vi "giveSolutionRubix.vi"() -> (1 "Commands to Execute":string[](array[string]))   [LabVIEW 2019]
uses:
  rubix solve code/Rubik's Solver.dll
panel:
  in  "RubixTab solver control":string[][](array[string])
  out "Loesung":i32[](array[numeric])
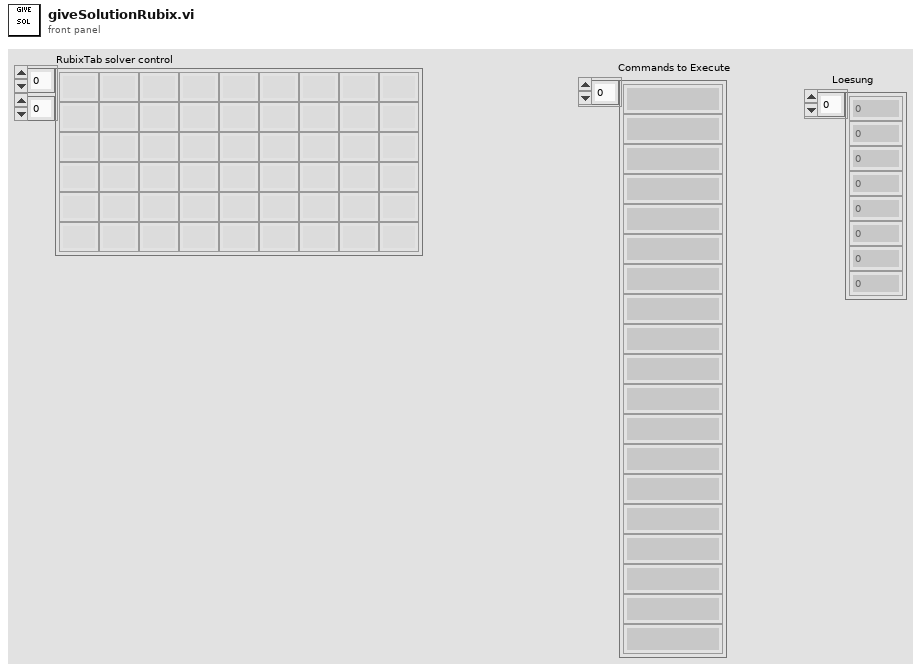
[diagram p1: front panel]
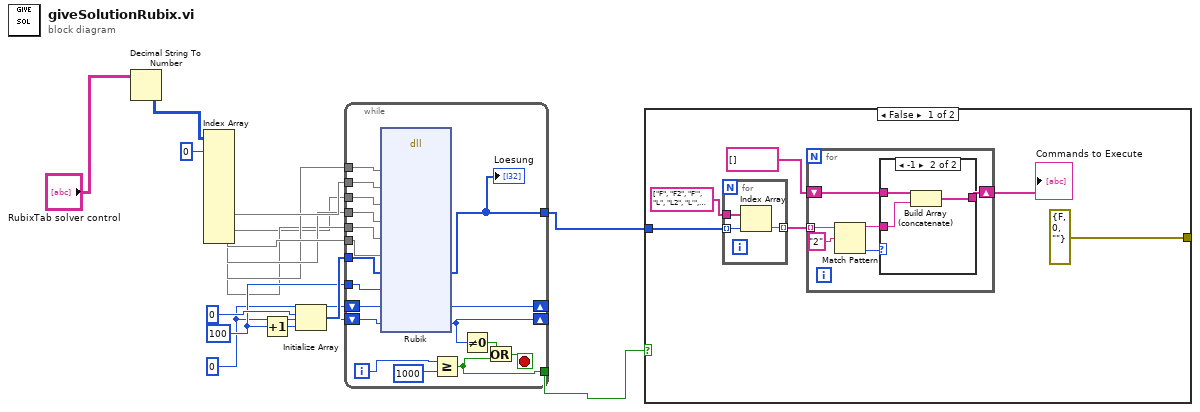
[diagram p0: block diagram]
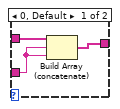
[diagram p2: hidden frame]
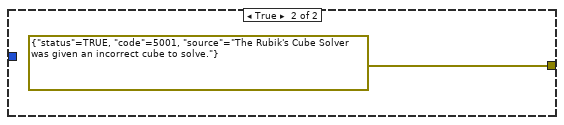
[diagram p3: hidden frame]
diagram:
  w12 = u8 0
  w13 = u16 100
  n1 = Decimal String To Number(string="RubixTab solver control") -> (number=w2:i32[][])  [unwired: 2 in, 1 out]
  n2 = Index Array(array=w2, index (row) #1=0 ("disabled index (col)")) -> (element #1=w10:i32[], element #2=w5:i32[], element #3=w9:i32[], element #4=w8:i32[], element #5=w7:i32[], element #6=w6:i32[])  [unwired: 11 in]
  n3 = Increment(x=w13) -> (x+1=w15:u16)
  n4 = Initialize Array(0 ("element"), w15) -> (w14:i32[])
  n5 = while {
    tunnel: w14 -> [w34]
    shift-right: [w18] -> _
    shift-left: w12 -> [w33]
    tunnel: w13 -> [w30]
    shift-right: [w31] -> _
    shift-left: w12 -> [w32]
    tunnel: [w23] -> w3
    tunnel: w7 -> [w29]
    tunnel: w10 -> [w28]
    tunnel: w5 -> [w27]
    tunnel: w8 -> [w26]
    tunnel: w6 -> [w25]
    tunnel: w9 -> [w24]
    tunnel: [w19] -> w4
    i -> [w22]
    stop <- w20 stop-if-true
    n6 = dll-call lib="D:/rubix/rubix solve code/Rubik's Solver.dll" fn="Rubik"("Up"=w29, "Front"=w28, "Right"=w27, "Left"=w26, "Down"=w25, "Back"=w24, "Loesung"=w34, "Anzahl"=w30, "Error"=w32, "ready"=w33) -> ("Loesung"=w23:i32[], "Error"=w31:u8, "ready"=w18:u8)  [unwired: 11 in, 2 out]
    "Loesung" <- w23
    n7 = Greater Or Equal?(x=w22, y=1000 ("x")) -> (x >= y?=w19:bool)
    n8 = Not Equal To 0?(x=w18) -> (x != 0?=w17:bool)
    n9 = Or(x=w17, y=w19) -> (x .or. y?=w20:bool)
  }
  n10 = case shown="False" w4 {
    tunnel: w3 -> [w38 _]
    tunnel: [errorcluster {"status"=FALSE, "code"=0, "source"=""} ("error IO") errorcluster {"status"=TRUE, "code"=5001, "source"="The Rubik's Cube Solver  was given an incorrect cube to solve."} ("error IO")] -> _
    frame False {
      n11 = for {
        tunnel: w38 -> [w55] mode=indexing
        tunnel: [w54] -> w40 mode=indexing
        tunnel: string[] ["F", "F2", "F'", "L", "L2", "L'", "U", "U2", "U'", "B", "B2", "B'", "R", "R2", "R'", "D", "D2", "D'"] -> [w53]
        n12 = Index Array(array=w53, index=w55) -> (element=w54:string)
      }
      n13 = for {
        tunnel: w40 -> [w46] mode=indexing
        shift-right: [w41] -> w36
        shift-left: string[] [] -> [w42]
        n14 = Match Pattern(string=w46, regular expression="2") -> (before substring=w43:string, offset past match=w44:i32)  [unwired: 1 in, 2 out]
        n15 = case shown="-1" w44 {
          tunnel: w43 -> [w47 w50]
          tunnel: w42 -> [w49 w52]
          tunnel: [w48 w51] -> w41
          frame 0, Default {
            n16 = Build Array (concatenate)(w49, w47, w47) -> (w48:string[])
          }
          frame -1 {
            n17 = Build Array (concatenate)(w52, w50) -> (w51:string[])
          }
        }
      }
      "Commands to Execute" <- w36
    }
    frame True {
    }
  }
